vi "DQMH_API_ReplyPayloadWindow.vi"() -> ()   [LabVIEW 2020]
doc: "_____\nCreated using Delacor QMH Event Scripter 5.0.0.106."
panel:
  out "ReplyData(Boolean)":bool
  # "Reply Payload Window"
  # "Instructions: Add controls to this panel. These controls will be added to the Reply Payload cluster for the new Request and Wait for Reply event. Use a descriptive label on each control.\n\nNote 1: There is no need to wrap the arguments with a cluster in this window. The Create New DQMH Event utility will take the controls in this VI and add them to an Reply Payload cluster when you are done. \n\nNote 2: You do not need to add an error cluster below... it will be created as part of the reply payload automatically."
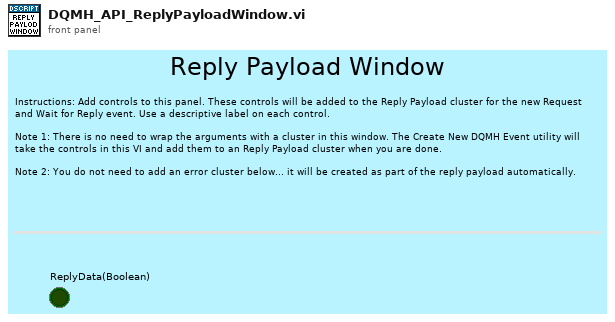
[diagram p1: front panel]
diagram:
